vi "autocoupler_v2.vi"() -> ()   [LabVIEW 2018]
uses:
  coupler_state.ctl
  <userlib>/PDamp/gain.ctl
  <userlib>/stepper/velocity settings.ctl
  <userlib>/stepper/travel limits.ctl
  <userlib>/PDamp/channel.ctl
panel:
  in  "zpos":dbl(slide)=394.2760942760943 scale=-10.0..10.0
  in  "ypos":dbl(slide)=394.2760942760943 scale=-30.0..30.0
  in  "x_fine_stepper":dbl(slide)=-26.599326599326588 caption="x_fine" scale=-50.0..50.0
  in  "x_course_stepper":dbl(slide)=394.2760942760943 caption="x_course" min=100.0 max=3900.0 scale=100.0..3900.0
  out "saved postion":sgl[][](array[numeric]) format="%_7g"
  in  "save position":bool
  out "Coupled":dbl=7.033088235294118
  out "Stray":dbl=7.259191176470588
  out "stepper_z_pos":dbl=2218.076171875 caption="z"
  out "stepper_y_pos":dbl=1867.105712890625 caption="y"
  out "stepper_x_pos":dbl=367.677001953125 caption="x"
  in  "stop":bool
  in  "abort":bool
  out "Cam":bool
  out "PD":bool
  out "Steppers":bool
  out "Piezos":bool
  out "State":T1=enum."stop"
  in  "settings tabn":T2(tab)
  in  "optimization tab":enum32{"Nelder-Mead"}(tab)
  out "simplex area":sgl[](graph)=[0.375, 0.1875, 0.10546875, 0.29516602, 0.51086426, 1.6301422, 1.6301422, 0.40753555, 0.12771606, 0.04718399, 0.11667609, 0.068683326, 0.068683326, 0.1192682, 0.1192682, 0.1192682, 0.1192682, 0.1192682, 0.04766251, 0.028668227, 0.016006902, 0.010568131, 0.003405895, 0.0014921137, 0.0014921074, 0.0014921074, 0.00037302685]
  out "Coupled intensity":dbl[](graph)=[0.8621323529411764, 1.340073585510254, 1.340073585510254, 1.340073585510254, 1.4430147409439087, 1.566176414489746, 3.8327205181121826, 3.8327205181121826, 3.8327205181121826, 3.8327205181121826, 3.8327205181121826, 4.630514621734619, 4.630514621734619, 4.630514621734619, 5.512867450714111, 5.878676414489746, 6.665441036224365, 6.665441036224365, 6.878676414489746, 6.917279243469238, 6.917279243469238, 6.954044342041016, 6.966911792755127, 6.966911792755127, 6.998161792755127, 7.042279243469238, 7.042279243469238, 7.042279243469238]
  out "current iteration":i32=26
  in  "settling time[ms]":u32=200
  in  "contraction/expansion\nparameters":T3={"expansion coefficient"=2.0, "contraction coefficient"=0.5, "shrink coefficient"=0.5}
  in  "max iterations":i32=100
  out "avpos":cluster{sgl[], sgl[]}(graph)
  in  "initial simplex":T4={"Initial size y[µm]"=3.0, "Initial size z[µm]"=1.0}
  in  "termination size":sgl=0.001
  out "ygrapg1":cluster{sgl[], dbl[]}(graph)={[1000.0, 1000.95215, 1003.7415, 1006.9983, 1011.278, 1016.626, 1022.976, 1030.3162, 1038.6584, 1048.0615, 1058.5583, 1069.9756, 1082.6392, 1096.0486, 1110.4932, 1126.0901, 1142.0935, 1157.992, 1174.0125, 1190.2563, 1206.1584, 1221.9861, 1238.031, 1253.8794, 1270.1099, 1286.2317, 1302.4512, 1318.0383, 1334.093, 1350.0513, 1365.9436, 1381.9299, 1397.8223, 1413.9478, 1429.79, 1445.7373, 1461.737, 1477.8247, 1493.9551, 1509.7705, 1525.6897, 1541.8323, 1557.688, 1573.7183, 1589.8083, 1605.7129, 1621.8115, 1637.948, 1653.5559, 1669.6423, 1685.6653, 1701.6772, 1717.7258, 1733.6426, 1749.9048, 1765.6921, 1782.0288, 1797.8796, 1814.0698, 1829.7119, 1845.8142, 1861.7993, 1878.0872, 1893.6365, 1909.729, 1925.6506, 1941.6064, 1957.5867, 1973.6548, 1989.5972, 2005.3746, 2021.6052, 2037.6587, 2053.5632, 2069.4531, 2085.6738, 2101.5442, 2117.5244, 2133.617, 2149.5447, 2165.3137, 2181.8408, 2197.472, 2213.3643, 2229.3225, 2245.404, 2261.4014, 2277.3328, 2293.385, 2309.4397, 2325.315, 2341.5076, 2357.2522, 2373.4534, 2389.6082, 2405.2454, 2421.432, 2437.317, 2453.0212, 2469.2456, 2485.2368, 2501.0999, 2517.0715, 2533.2825, 2549.159, 2565.0476, 2581.0107, 2596.8494, 2613.0505, 2628.894, 2645.0586, 2661.001, 2676.9934, 2692.8577, 2708.8953, 2724.795, 2741.2122, 2756.858, 2772.865, 2788.9014, 2804.7375, 2820.7458, 2836.7175, 2852.915, 2868.7244, 2884.5178, 2899.3396, 2913.424, 2926.0327, 2937.7893, 2948.5083, 2958.5083, 2966.9885, 2974.7607, 2981.333, 2987.0557, 2991.665, 2995.2612, 2997.8699, 2999.4556], [7.983455882352941, 7.9724264705882355, 7.948529411764706, 7.9099264705882355, 7.849264705882353, 7.783088235294118, 7.735294117647059, 7.731617647058823, 7.825367647058823, 8.001838235294118, 8.117647058823529, 8.060661764705882, 8.084558823529411, 8.314338235294118, 8.625, 8.5, 8.472426470588236, 8.466911764705882, 8.465073529411764, 8.463235294117647, 8.461397058823529, 8.485294117647058, 8.492647058823529, 8.505514705882353, 8.439338235294118, 8.380514705882353, 8.306985294117647, 8.15625, 7.954044117647059, 7.783088235294118, 7.731617647058823, 7.762867647058823, 7.7849264705882355, 7.645220588235294, 7.610294117647059, 7.47610294117647, 7.161764705882353, 6.790441176470588, 6.492647058823529, 6.301470588235294, 6.1599264705882355, 6.1911764705882355, 6.080882352941177, 5.658088235294118, 5.461397058823529, 5.0036764705882355, 4.075367647058823, 3.0588235294117645, 2.0643382352941178, 1.349264705882353, 0.9172794117647058, 0.65625, 0.5110294117647058, 0.4411764705882353, 0.40625, 0.3860294117647059, 0.3676470588235294, 0.3676470588235294, 0.33088235294117646, 0.3290441176470588, 0.33455882352941174, 0.34191176470588236, 0.3639705882352941, 0.40808823529411764, 0.5588235294117647, 0.4430147058823529, 0.4944852941176471, 0.5422794117647058, 0.6213235294117647, 0.8088235294117647, 1.2610294117647058, 2.145220588235294, 3.6966911764705883, 5.827205882352941, 8.349264705882353, 10.806985294117647, 12.606617647058822, 13.707720588235293, 14.474264705882353, 15.262867647058822, 16.009191176470587, 16.470588235294116, 16.795955882352942, 17.18198529411765, 17.490808823529413, 17.626838235294116, 17.797794117647058, 18.020220588235293, 18.110294117647058, 18.198529411764707, 18.34375, 18.43566176470588, 18.441176470588236, 18.49448529411765, 18.49264705882353, 18.450367647058822, 18.43198529411765, 18.36764705882353, 18.314338235294116, 18.28125, 18.21875, 18.18014705882353, 18.176470588235293, 18.141544117647058, 18.11764705882353, 18.090073529411764, 18.097426470588236, 18.08639705882353, 18.051470588235293, 18.049632352941178, 18.06801470588235, 18.08639705882353, 18.112132352941178, 18.13051470588235, 18.143382352941178, 18.15441176470588, 18.15625, 18.159926470588236, 18.16360294117647, 18.178308823529413, 18.125, 18.115808823529413, 18.110294117647058, 18.080882352941178, 18.06801470588235, 18.064338235294116, 18.06801470588235, 18.080882352941178, 18.095588235294116, 18.10110294117647, 18.104779411764707, 18.106617647058822, 18.108455882352942, 18.14889705882353, 18.172794117647058, 18.176470588235293, 18.18014705882353, 18.183823529411764, 18.18198529411765, 18.18566176470588]}
  in  "initial_align":bool
  in  "z_scan_params":T5={"-offset"=100.0, "+offset"=500.0, "speed"=0.05, "threshold"=4.0, "y-offset"=0.0}
  in  "scan_y_params":T6={"startPos"=1000.0, "endPos"=3000.0, "speed"=1.0, "threshold"=1.0} {"endPos" min=0 max=4000; "startPos" min=0 max=4000}
  out "ygraph2":cluster{sgl[], dbl[]}(graph)={[1685.6653, 1686.499, 1688.3215, 1691.1292, 1694.1357, 1697.3169, 1700.5322, 1704.1016, 1708.3813, 1713.4692, 1716.6699, 1719.8682, 1723.0444, 1726.2427, 1729.4495, 1732.5269, 1735.697, 1738.8977, 1742.3877, 1745.6311, 1748.7732, 1751.9434, 1755.1404, 1758.3447, 1761.2573, 1764.436, 1767.6306, 1770.8411, 1774.0405, 1777.2473, 1780.6677, 1783.8635, 1787.0642, 1790.2393, 1793.479, 1796.676, 1799.6301, 1802.8064, 1806.0144, 1809.6118, 1812.815, 1815.9985, 1820.2808, 1825.3357, 1828.5254, 1831.7236, 1834.7595, 1837.959, 1841.1719, 1844.6936, 1847.8674, 1851.0742, 1854.2603, 1857.4609, 1860.6201, 1863.5168, 1866.7432, 1869.9121, 1874.6008, 1879.5203, 1882.9688, 1886.1768, 1889.3848, 1892.5635, 1895.7739, 1898.9429, 1901.8823, 1905.0769, 1908.2776, 1911.5027, 1914.685, 1917.8589, 1921.0779, 1924.646, 1928.9673, 1934.0332, 1937.2205, 1940.2246, 1943.4375, 1946.637, 1950.1782, 1954.602, 1959.751, 1962.9431, 1965.8203, 1969.0149, 1972.2168, 1975.4163, 1978.6108, 1981.8384, 1985.2454, 1987.7124, 1989.1687], [8.908088235294118, 8.935661764705882, 8.970588235294118, 8.996323529411764, 8.79595588235294, 8.994485294117647, 9.262867647058824, 9.323529411764707, 9.196691176470589, 9.384191176470589, 9.134191176470589, 9.169117647058824, 8.48345588235294, 8.503676470588236, 8.98345588235294, 9.20220588235294, 9.806985294117647, 10.07720588235294, 10.033088235294118, 10.148897058823529, 10.196691176470589, 10.238970588235293, 10.193014705882353, 10.1875, 10.13970588235294, 10.134191176470589, 10.126838235294118, 10.136029411764707, 10.169117647058824, 10.266544117647058, 10.373161764705882, 10.488970588235293, 10.680147058823529, 10.775735294117647, 10.85845588235294, 10.904411764705882, 10.875, 10.726102941176471, 10.455882352941176, 10.04595588235294, 9.220588235294118, 8.415441176470589, 7.50735294117647, 6.466911764705882, 5.525735294117647, 4.7775735294117645, 3.9301470588235294, 3.332720588235294, 2.625, 2.422794117647059, 2.4761029411764706, 3.0386029411764706, 2.479779411764706, 2.5533088235294117, 3.7279411764705883, 3.8731617647058822, 3.9871323529411766, 4.261029411764706, 5.665441176470588, 7.85110294117647, 9.647058823529411, 11.189338235294118, 13.503676470588236, 14.92095588235294, 17.13235294117647, 18.18014705882353, 19.69301470588235, 20.227941176470587, 21.159926470588236, 21.36948529411765, 21.641544117647058, 21.626838235294116, 21.360294117647058, 21.051470588235293, 20.65073529411765, 20.207720588235293, 19.996323529411764, 19.88051470588235, 19.81985294117647, 19.81066176470588, 19.84926470588235, 19.983455882352942, 20.06801470588235, 20.1875, 20.170955882352942, 20.11948529411765, 20.027573529411764, 19.928308823529413, 19.823529411764707, 19.68566176470588, 19.597426470588236, 19.509191176470587, 19.479779411764707]}
  out "zgraph":cluster{sgl[], dbl[]}(graph)={[2142.5427, 2143.4863, 2144.281, 2145.0757, 2145.8716, 2146.6602, 2147.4707, 2148.2068, 2149.0112, 2149.8047, 2150.5933, 2151.3916, 2152.1948, 2152.9944, 2153.7927, 2154.5813, 2155.3857, 2156.1816, 2156.98, 2157.782, 2158.5815, 2159.3774, 2160.2686, 2161.0657, 2161.8652, 2162.9053, 2163.7036, 2164.497, 2165.3088, 2166.0999, 2166.8933, 2167.6953, 2168.4949, 2169.292, 2170.094, 2170.8984, 2171.6907, 2172.5012, 2173.2947, 2174.0894, 2174.889, 2175.6982, 2176.488, 2177.295, 2178.0872, 2178.8953, 2179.6838, 2180.4968, 2181.7615, 2182.5537, 2183.3557, 2184.1516, 2184.95, 2185.8423, 2186.599, 2187.3462, 2188.2385, 2189.0369, 2189.8352, 2190.89, 2192.146, 2192.948, 2193.7402, 2194.535, 2195.4224, 2196.2134, 2196.958, 2198.0737, 2199.3347, 2200.1343, 2200.9424, 2201.7346, 2202.5317, 2203.335, 2204.1907, 2204.995, 2205.797, 2206.5967, 2207.384, 2208.186, 2208.933, 2209.735, 2210.536, 2211.3318, 2212.223, 2213.0322, 2213.8257, 2214.6155, 2215.4236, 2216.1328, 2216.9214, 2218.0762], [26.39889705882353, 26.501838235294116, 26.566176470588236, 26.488970588235293, 26.5, 26.46875, 26.422794117647058, 26.52941176470588, 26.393382352941178, 26.308823529411764, 26.386029411764707, 26.33639705882353, 26.43566176470588, 26.483455882352942, 26.308823529411764, 26.356617647058822, 26.338235294117645, 26.330882352941178, 26.488970588235293, 26.358455882352942, 26.3125, 26.463235294117645, 26.419117647058822, 26.551470588235293, 26.454044117647058, 26.27941176470588, 26.369485294117645, 26.31801470588235, 26.420955882352942, 26.47426470588235, 26.240808823529413, 26.33639705882353, 26.27389705882353, 26.220588235294116, 26.28676470588235, 26.03676470588235, 25.94485294117647, 26.165441176470587, 26.06801470588235, 26.209558823529413, 26.19301470588235, 25.863970588235293, 26.090073529411764, 26.169117647058822, 26.266544117647058, 26.387867647058822, 26.020220588235293, 26.06066176470588, 26.323529411764707, 26.159926470588236, 26.240808823529413, 25.928308823529413, 25.983455882352942, 26.28860294117647, 26.0625, 26.09191176470588, 25.71139705882353, 25.441176470588236, 25.753676470588236, 25.431985294117645, 25.53676470588235, 24.981617647058822, 25.18566176470588, 25.41360294117647, 24.875, 24.946691176470587, 24.71691176470588, 24.60110294117647, 25.290441176470587, 24.928308823529413, 25.544117647058822, 25.137867647058822, 25.270220588235293, 26.06985294117647, 25.21139705882353, 25.733455882352942, 25.884191176470587, 25.207720588235293, 27.90625, 26.965073529411764, 24.926470588235293, 28.25, 26.625, 24.78125, 22.27941176470588, 15.957720588235293, 16.490808823529413, 19.59191176470588, 17.606617647058822, 12.955882352941176, 8.367647058823529, 3.6011029411764706]}
  out "y_out":sgl=1837.1057
  out "z_out":sgl=2218.0762
  in  "stepsize x":i32
  in  "HWSerialNum x":i32=90897056 caption="serial nr"
  in  "HWSerialNum y":i32=90897057 caption="serial nr"
  in  "HWSerialNum z":i32=90897058 caption="serial nr"
  in  "MG17Motor y":refnum<k7>(container)
  in  "MG17Motor x":refnum<k7>(container)
  in  "MG17Motor z":refnum<k7>(container)
  in  "z_0":dbl=394.2760942760943 caption="z0" min=100.0 max=3900.0
  in  "y_0":dbl=394.2760942760943 caption="y0" min=100.0 max=3900.0
  in  "piezo_z_setmiddle":bool
  in  "piezo_y_setmiddle":bool
  in  "piezo_x_setmiddle":bool
  in  "x-axis":refnum<k7>(container)
  in  "y-axis":refnum<k7>(container)
  in  "z-axis":refnum<k7>(container)
  in  "serial number x":i32=91897094 caption="serial nr"
  in  "srl nr y-axis":i32=91897095 caption="serial nr"
  in  "srl nr z-axis":i32=91897096 caption="serial nr"
  in  "Change_cam_settings":bool
  out "Cam Info":T7={"Model"="IDS GmbH", "Camera ID"="UI124xSE-M", "Firmware"=""}
  in  "Camera ID":i32
  in  "Exposure[ms]":dbl=9.999750247413404 format="%#_13g"
  in  "camera live":bool=TRUE
  in  "ROI":T8={"posX"=0, "posY"=0, "Width"=1280, "height"=1024}
  out "ROI_current":T8
  in  "PD_comport":refnum<visa-resource-name>="COM4"
  out "status":string="rdy\r\n"
  in  "gain":T9=enum."1"
  in  "optimize":bool
  in  "stepper_home":bool
  in  "piezo_home":bool
  out "image":u8[][](graph)
  # "current position"
  # "x-axis"
  # "y-axis"
  # "z-axis"
  # "x-axis"
  # "y-axis"
  # "z-axis"
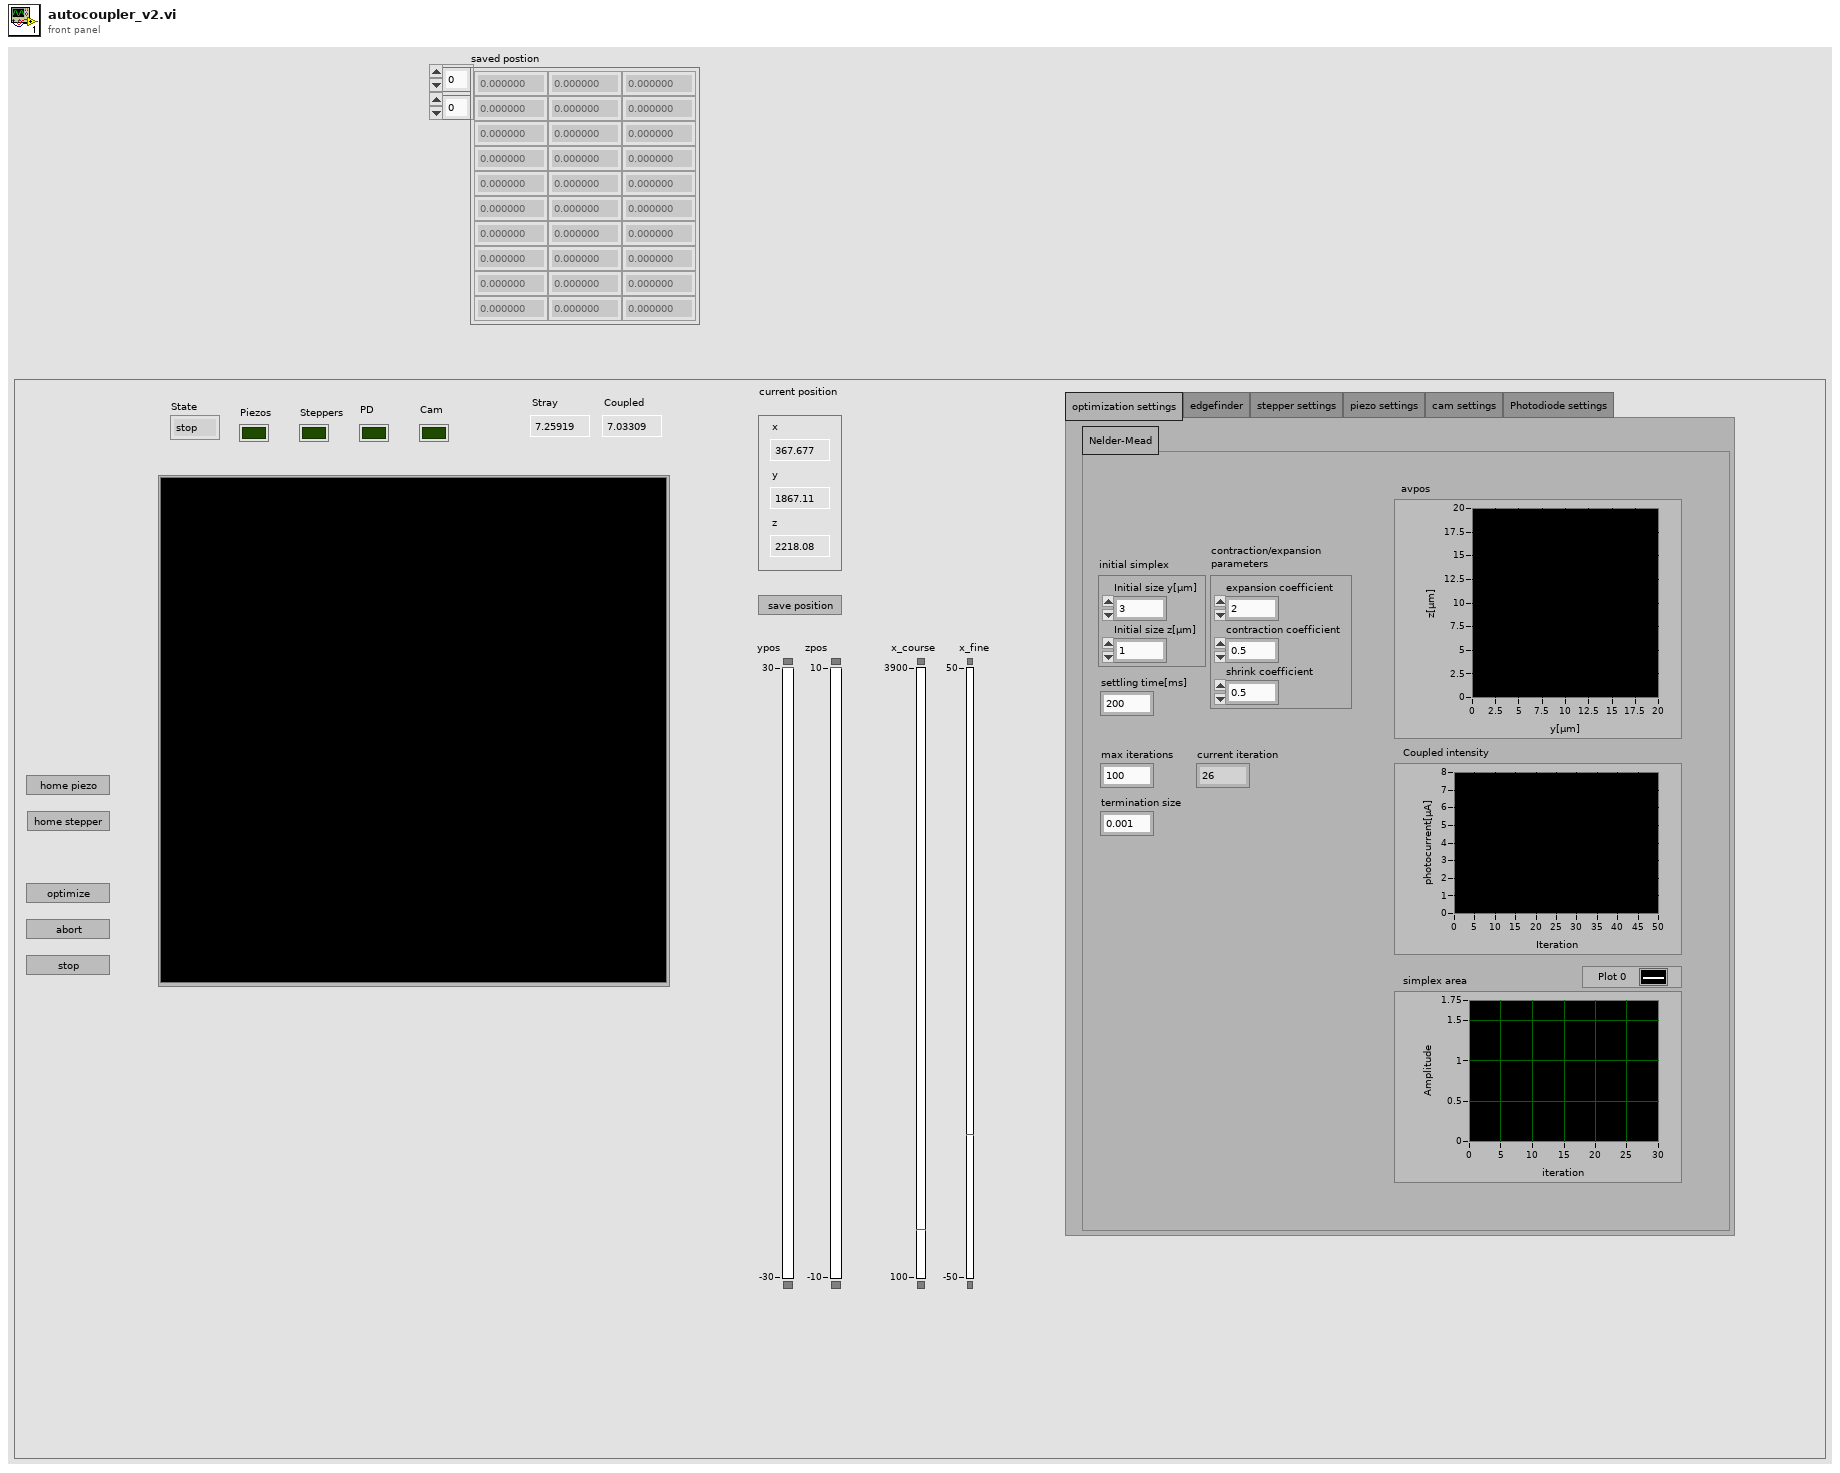
[diagram p1: front panel]
types:
  T1 = typedef "coupler_state.ctl" = enum16{"init", "idle", "zero_steppers", "zero_piezo", "edge_find", "save_position", "optimize", "stop", "error"}
  T2 = enum32{"optimization settings", "edgefinder", "stepper settings", "piezo settings", "cam settings", "Photodiode settings"}
  T3 = cluster{"expansion coefficient":dbl, "contraction coefficient":dbl, "shrink coefficient":dbl}
  T4 = cluster{"Initial size y[µm]":sgl, "Initial size z[µm]":sgl}
  T5 = cluster{"-offset":sgl, "+offset":sgl, "speed":sgl, "threshold":dbl, "y-offset":dbl}
  T6 = cluster{"startPos":sgl, "endPos":sgl, "speed":sgl, "threshold":sgl}
  T7 = cluster{"Model":string, "Camera ID":string, "Firmware":string}
  T8 = cluster{"posX":i32, "posY":i32, "Width":i32, "height":i32}
  T9 = typedef "gain.ctl" = enum16{"2/3", "1", "2", "4", "8", "16"}
  T10 = typedef "velocity settings.ctl" = cluster{"pfMinVel":sgl, "pfAccn":sgl, "pfMaxVel":sgl}
  T11 = typedef "channel.ctl" = enum16{"ch1", "ch2", "ch3", "ch4"}
  T12 = typedef "travel limits.ctl" = cluster{"pfRevPosLimit":sgl, "pfFwdPosLimit":sgl, "plLimitMode":i32}
  T13 = typedef "PDref.ctl" = cluster{"PD Reference":refnum<visa-resource-name>, "conversrion gain":dbl}
  T14 = cluster{"reference out":refnum<k7>, "reference out":refnum<k7>, "reference out":refnum<k7>}
  T15 = cluster{"reference out":refnum<k24>, "PDcluster":T13, cluster{"reference out":refnum<k7>, "reference out":refnum<k7>, "reference out":refnum<k7>}, cluster{"reference out":refnum<k7>, "reference out":refnum<k7>, "reference out":refnum<k7>}}
  T16 = cluster{"Reflected":sgl[][], "Expanded":sgl[][], "Contracted inside":sgl[][], "Contracted outside":sgl[][], "Shrunk":sgl[][]}
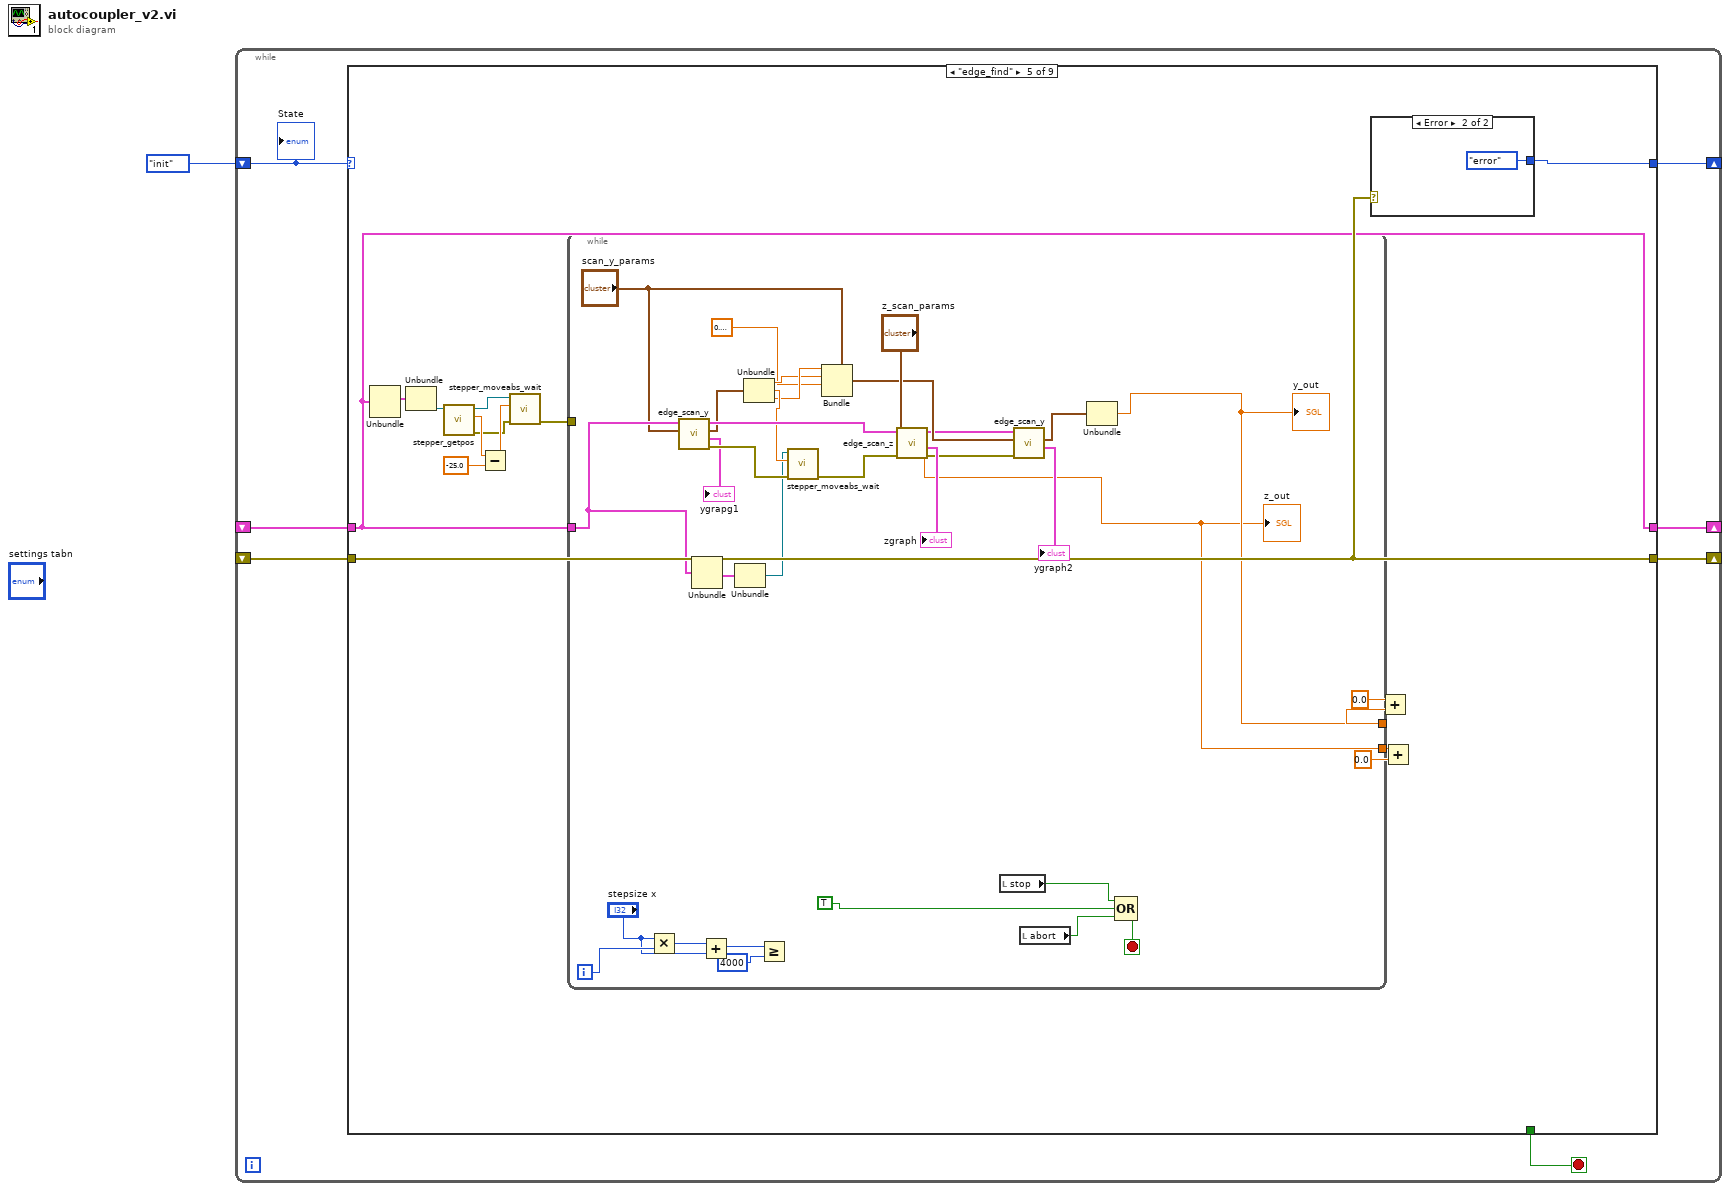
[diagram p0: block diagram]
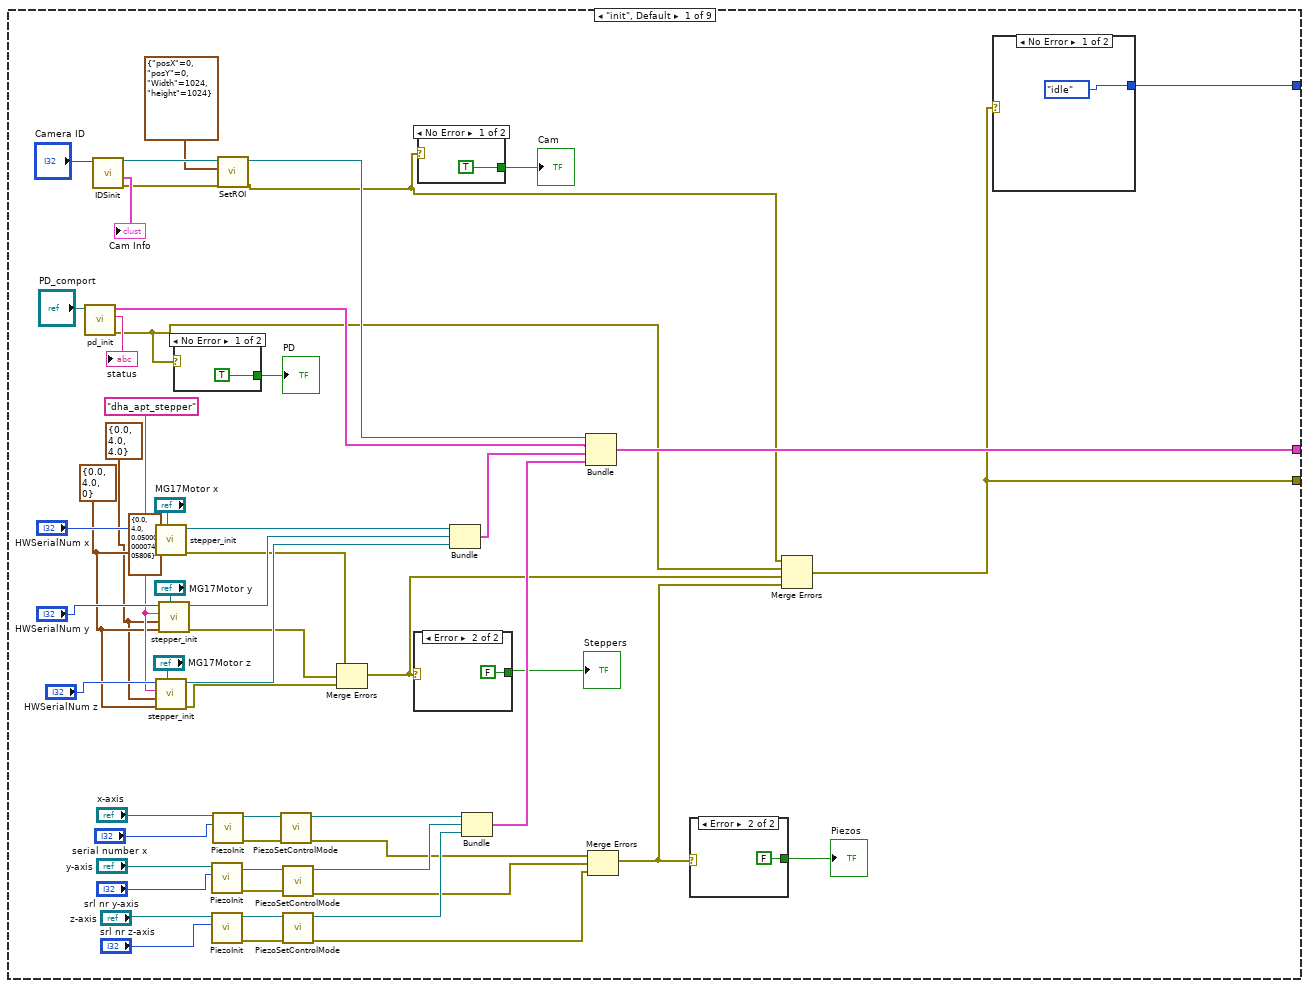
[diagram p2: hidden frame]
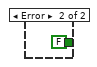
[diagram p3: hidden frame]
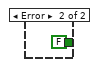
[diagram p4: hidden frame]
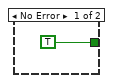
[diagram p5: hidden frame]
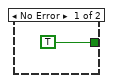
[diagram p6: hidden frame]
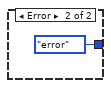
[diagram p7: hidden frame]
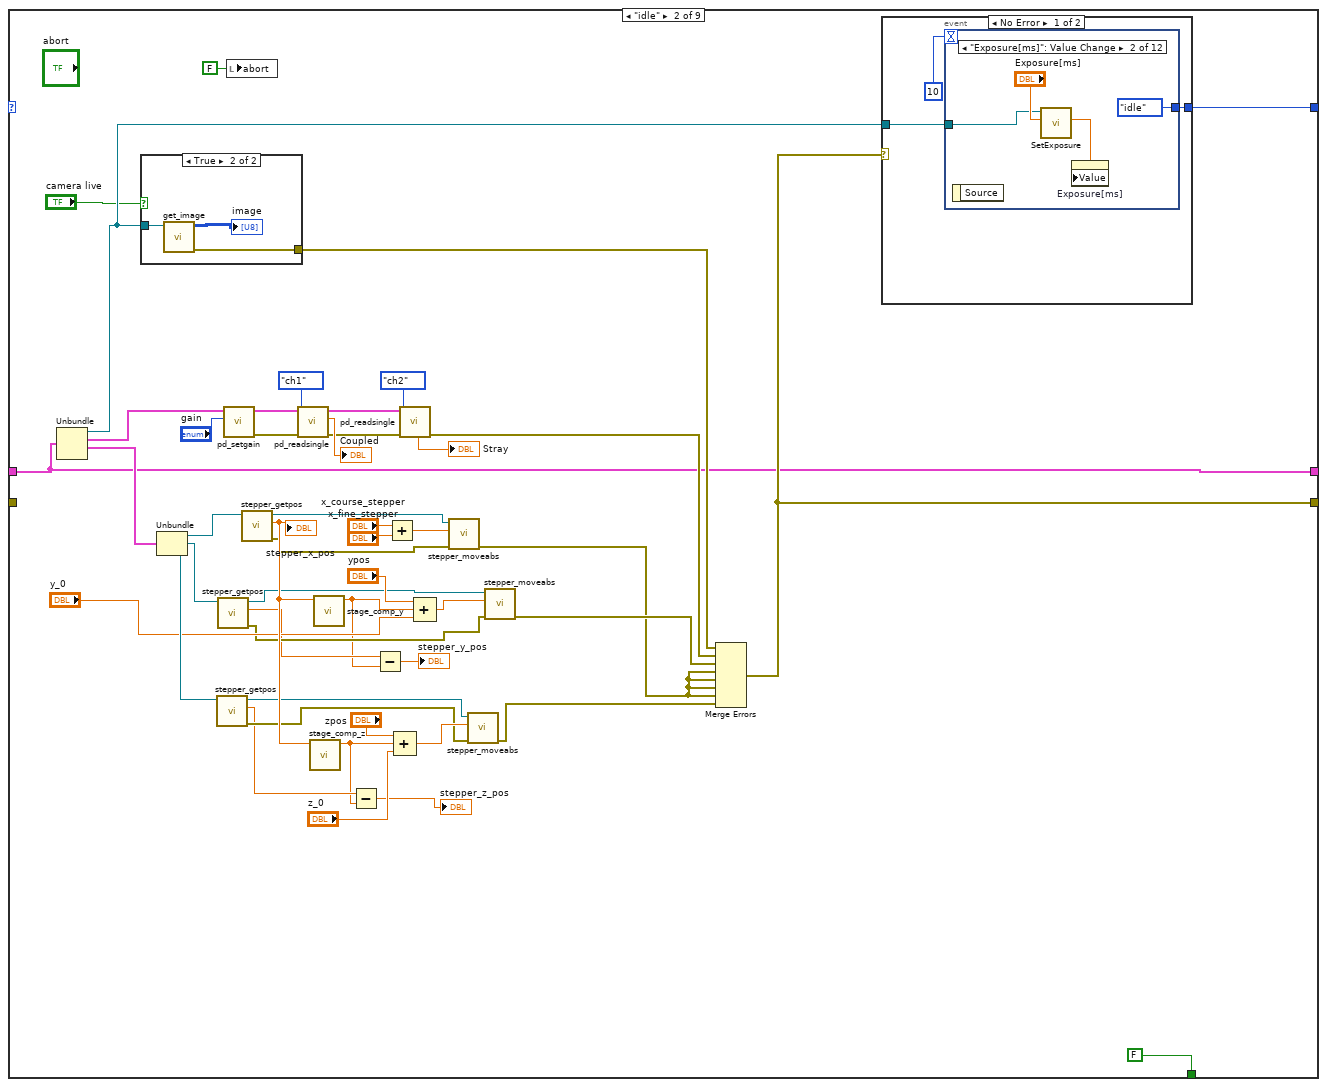
[diagram p8: hidden frame]
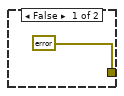
[diagram p9: hidden frame]
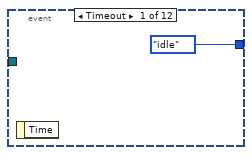
[diagram p10: hidden frame]
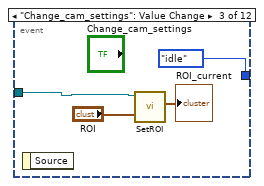
[diagram p11: hidden frame]
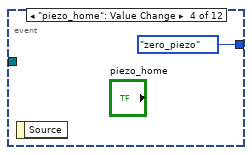
[diagram p12: hidden frame]
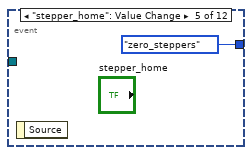
[diagram p13: hidden frame]
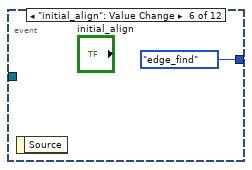
[diagram p14: hidden frame]
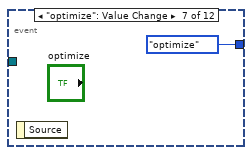
[diagram p15: hidden frame]
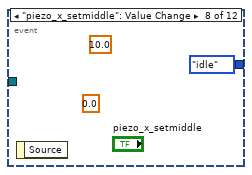
[diagram p16: hidden frame]
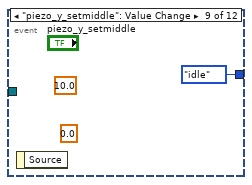
[diagram p17: hidden frame]
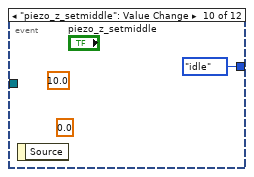
[diagram p18: hidden frame]
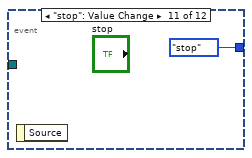
[diagram p19: hidden frame]
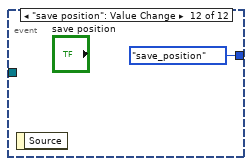
[diagram p20: hidden frame]
diagram:
  n1 = while {
    shift-right: [w7] -> _
    shift-left: coupler_state."init" -> [w8]
    shift-right: [w6] -> _
    shift-left: _ -> [w5]
    shift-right: [w3] -> _
    shift-left: _ -> [w2]
    stop <- w4 stop-if-true
    n2 = case shown="\"edge_find\"" w8 {
      tunnel: [w30 w122 w151 w170 w187 w245 w252 w318 w321] -> w7
      tunnel: [w31 w100 w150 w162 w185 w243 w251 w308 w331] -> w6
      tunnel: w5 -> [_ w100 w150 w162 w185 w243 w251 w308 w331]
      tunnel: [_ FALSE _ _ _ _ _ TRUE _] -> w4
      tunnel: [w11 w106 w149 w161 w186 w244 w249 w306 w322] -> w3
      tunnel: w2 -> [_ _ _ _ w186 w244 w250 w306 w323]
      frame "init", Default {
        w42 = T12 {"pfRevPosLimit"=0.0, "pfFwdPosLimit"=4.0, "plLimitMode"=0} ("travel limits")
        w10 = T10 {"pfMinVel"=0.0, "pfAccn"=4.0, "pfMaxVel"=4.0} ("velocity parameters")
        w43 = "dha_apt_stepper" ("parameter set")
        n3 = call <userlib>:"pd_init.vi"("VISA resource name"="PD_comport") -> ("error out"=w13:errorcluster, "status"=→"status":string, "PDcluster"=w32:T13)  [unwired: 8 in]
        n4 = call <userlib>:"IDSinit.vi"("Camera ID"="Camera ID") -> ("error out"=w17:errorcluster, "Cam Info"=→"Cam Info":T7, "reference out"=w29:refnum<k24>)  [unwired: 6 in, 1 out]
        n5 = call <userlib>:"stepper_init.vi"("MG17Motor"="MG17Motor x", "travel limits"=w42, "velocity parameters"=T10 {"pfMinVel"=0.0, "pfAccn"=4.0, "pfMaxVel"=0.05}, "parameter set"=w43, "HWSerialNum"="HWSerialNum x") -> ("error out"=w20:errorcluster, "reference out"=w39:refnum<k7>)  [unwired: 3 in, 2 out]
        n6 = call <userlib>:"stepper_init.vi"("MG17Motor"="MG17Motor z", "travel limits"=w42, "velocity parameters"=w10, "parameter set"=w43, "HWSerialNum"="HWSerialNum z") -> ("error out"=w22:errorcluster, "reference out"=w41:refnum<k7>)  [unwired: 3 in, 2 out]
        n7 = call <userlib>:"stepper_init.vi"("MG17Motor"="MG17Motor y", "travel limits"=w42, "velocity parameters"=w10, "parameter set"=w43, "HWSerialNum"="HWSerialNum y") -> ("error out"=w21:errorcluster, "reference out"=w40:refnum<k7>)  [unwired: 3 in, 2 out]
        n8 = case shown="No Error" w13 {
          tunnel: [TRUE ("Piezos") FALSE ("Piezos")] -> w18
          frame No Error {
          }
          frame Error {
          }
        }
        "PD" <- w18
        n9 = call <userlib>:"PiezoInit.vi"("reference"="y-axis", "HWSerialNum"="srl nr y-axis") -> ("reference out"=w56:refnum<k7>, "error out"=w54:errorcluster)  [unwired: 7 in]
        n10 = call <userlib>:"PiezoInit.vi"("reference"="z-axis", "HWSerialNum"="srl nr z-axis") -> ("reference out"=w57:refnum<k7>, "error out"=w53:errorcluster)  [unwired: 7 in]
        n11 = call <userlib>:"PiezoInit.vi"("reference"="x-axis", "HWSerialNum"="serial number x") -> ("reference out"=w58:refnum<k7>, "error out"=w55:errorcluster)  [unwired: 7 in]
        n12 = call <userlib>:"SetROI.vi"("error in (no error)"=w17, "SizeIn"=T8 {"posX"=0, "posY"=0, "Width"=1024, "height"=1024}, "reference in"=w29) -> ("error out"=w12:errorcluster, "reference out"=w27:refnum<k24>)  [unwired: 5 in, 1 out]
        n13 = call <userlib>:"PiezoSetControlMode.vi"("error in (no error)"=w55, "reference"=w58) -> ("error out"=w26:errorcluster, "reference out"=w50:refnum<k7>)  [unwired: 8 in]
        n14 = call <userlib>:"PiezoSetControlMode.vi"("error in (no error)"=w54, "reference"=w56) -> ("error out"=w25:errorcluster, "reference out"=w51:refnum<k7>)  [unwired: 8 in]
        n15 = call <userlib>:"PiezoSetControlMode.vi"("error in (no error)"=w53, "reference"=w57) -> ("error out"=w24:errorcluster, "reference out"=w52:refnum<k7>)  [unwired: 8 in]
        n16 = Merge Errors(w20, w21, w22) -> (w14:errorcluster)
        n17 = case shown="Error" w14 {
          tunnel: [TRUE ("Piezos") FALSE ("Piezos")] -> w19
          frame No Error {
          }
          frame Error {
          }
        }
        "Steppers" <- w19
        n18 = case shown="No Error" w12 {
          tunnel: [TRUE ("Piezos") FALSE ("Piezos")] -> w16
          frame No Error {
          }
          frame Error {
          }
        }
        "Cam" <- w16
        n19 = Bundle("reference out"=w39, "reference out"=w40, "reference out"=w41) -> (w33:T14)  [unwired: 1 in]
        n20 = Bundle("reference out"=w50, "reference out"=w51, "reference out"=w52) -> (w34:T14)  [unwired: 1 in]
        n21 = Bundle("reference out"=w27, "PDcluster"=w32, w33, w34) -> (w31:T15)  [unwired: 1 in]
        n22 = Merge Errors(w26, w25, w24) -> (w15:errorcluster)
        n23 = case shown="Error" w15 {
          tunnel: [TRUE ("Piezos") FALSE ("Piezos")] -> w23
          frame No Error {
          }
          frame Error {
          }
        }
        "Piezos" <- w23
        n24 = Merge Errors(w12, w13, w14, w15) -> (w11:errorcluster)
        n25 = case shown="No Error" w11 {
          tunnel: [coupler_state."idle" coupler_state."error"] -> w30
          frame No Error {
          }
          frame Error {
          }
        }
      }
      frame "idle" {
        n26 = Unbundle(w100) -> ("reference out"=w103:refnum<k24>, "PDcluster"=w121:T13, w110:T14)  [unwired: 1 out]
        n27 = case shown="True" "camera live" {
          tunnel: [errorcluster {"status"=FALSE, "code"=0, "source"=""} ("error out") w125] -> w104
          tunnel: w103 -> [_ w124]
          frame False {
          }
          frame True {
            n28 = call <userlib>:"get_image.vi"("reference"=w124) -> ("error out"=w125:errorcluster, "Array"=→"image":u8[][])  [unwired: 9 in]
          }
        }
        n29 = Unbundle(w110) -> ("reference out"=w113:refnum<k7>, "reference out"=w112:refnum<k7>, "reference out"=w111:refnum<k7>)
        n30 = call <userlib>:"stepper_getpos.vi"("reference"=w111) -> ("error out"=w85:errorcluster, "pfPosition[µm]"=w78:sgl, "reference out"=w91:refnum<k7>)  [unwired: 8 in]
        n31 = call <userlib>:"stepper_getpos.vi"("reference"=w112) -> ("error out"=w83:errorcluster, "pfPosition[µm]"=w76:sgl, "reference out"=w88:refnum<k7>)  [unwired: 8 in]
        n32 = call <userlib>:"pd_setgain.vi"("gain"="gain", "PDcluster in"=w121) -> ("error out"=w108:errorcluster, "PDcluster out"=w119:T13)  [unwired: 7 in, 1 out]
        n33 = local write "abort"(FALSE ("abort")) -> ()
        n34 = call <userlib>:"stepper_getpos.vi"("reference"=w113) -> ("error out"=w81:errorcluster, "pfPosition[µm]"=w95:sgl, "reference out"=w96:refnum<k7>)  [unwired: 8 in]
        "stepper_x_pos" <- w95
        n35 = call <userlib>:"pd_readsingle.vi"("PDcluster in"=w119, "channel"=channel."ch1", "error in (no error)"=w108) -> ("PDcluster out"=w117:T13, "photocurrent"=→"Coupled":dbl, "error out"=w107:errorcluster)  [unwired: 5 in]
        n36 = call "stage_comp_z.vi"("xpos"=w95) -> ("zcorr"=w77:dbl)  [unwired: 10 in]
        n37 = call "stage_comp_y.vi"("xpos"=w95) -> ("ycorr"=w75:dbl)  [unwired: 9 in, 1 out]
        n38 = Subtract(x=w78, y=w77) -> (x-y=→"stepper_z_pos":dbl)
        n39 = Subtract(x=w76, y=w75) -> (x-y=→"stepper_y_pos":dbl)
        n40 = Add(x="x_course_stepper", y="x_fine_stepper") -> (x+y=w97:dbl)
        n41 = Compound Arithmetic op=ADD("zpos", w77, "z_0") -> (w92:dbl)
        n42 = call <userlib>:"pd_readsingle.vi"("PDcluster in"=w117, "channel"=channel."ch2", "error in (no error)"=w107) -> ("photocurrent"=→"Stray":dbl, "error out"=w105:errorcluster)  [unwired: 5 in, 1 out]
        n43 = Compound Arithmetic op=ADD("ypos", w75, "y_0") -> (w79:dbl)
        n44 = call <userlib>:"stepper_moveabs.vi"("error in (no error)"=w81, "fAbsPos[µm]"=w97, "reference"=w96) -> ("error out"=w80:errorcluster)  [unwired: 7 in, 1 out]
        n45 = call <userlib>:"stepper_moveabs.vi"("error in (no error)"=w85, "fAbsPos[µm]"=w92, "reference"=w91) -> ("error out"=w84:errorcluster)  [unwired: 7 in, 1 out]
        n46 = call <userlib>:"stepper_moveabs.vi"("error in (no error)"=w83, "fAbsPos[µm]"=w79, "reference"=w88) -> ("error out"=w82:errorcluster)  [unwired: 7 in, 1 out]
        n47 = Merge Errors(w104, w105, w82, w80, w80, w80, w80, w84) -> (w106:errorcluster)
        n48 = case shown="No Error" w106 {
          tunnel: [w128 coupler_state."error"] -> w122
          tunnel: w103 -> [w127 _]
          frame No Error {
            n49 = event shown="[1] \"Exposure[ms]\": Value Change" {
              selector: _ -> [_ _ _ _ _ _ _ _ _ _ _ _]
              dyn-events: _ -> [_ _ _ _ _ _ _ _ _ _ _ _]
              timeout: 10 -> [_ _ _ _ _ _ _ _ _ _ _ _]
              tunnel: [coupler_state."idle" coupler_state."idle" coupler_state."idle" coupler_state."zero_piezo" coupler_state."zero_steppers" coupler_state."edge_find" coupler_state."optimize" coupler_state."idle" coupler_state."idle" coupler_state."idle" coupler_state."stop" coupler_state."save_position"] -> w128
              tunnel: w127 -> [_ w132 w137 _ _ _ _ _ _ _ _ _]
              event Timeout {
                n50 = event-data() -> ()  [unwired: 1 in, 1 out]
              }
              event "Exposure[ms]": Value Change {
                n51 = event-data() -> ()  [unwired: 1 in, 1 out]
                n52 = call <userlib>:"SetExposure.vi"("Exposure[ms]"="Exposure[ms]", "Reference in"=w132) -> ("exposure"=w133:dbl)  [unwired: 5 in, 3 out]
                n53 = property on="Exposure[ms]" class="DigNum (strict)"("Value"=w133) -> ()  [unwired: 2 in, 2 out]
              }
              event "Change_cam_settings": Value Change {
                n54 = event-data() -> ()  [unwired: 1 in, 1 out]
                n55 = call <userlib>:"SetROI.vi"("SizeIn"="ROI", "reference in"=w137) -> ("SizeOut"=→"ROI_current":T8)  [unwired: 6 in, 2 out]
              }
              event "piezo_home": Value Change {
                n56 = event-data() -> ()  [unwired: 1 in, 1 out]
              }
              event "stepper_home": Value Change {
                n57 = event-data() -> ()  [unwired: 1 in, 1 out]
              }
              event "initial_align": Value Change {
                n58 = event-data() -> ()  [unwired: 1 in, 1 out]
              }
              event "optimize": Value Change {
                n59 = event-data() -> ()  [unwired: 1 in, 1 out]
              }
              event "piezo_x_setmiddle": Value Change {
                (unwired) 0.0 ("z_fine_piezo")
                (unwired) 10.0 ("x_course_piezo")
                n60 = event-data() -> ()  [unwired: 1 in, 1 out]
              }
              event "piezo_y_setmiddle": Value Change {
                (unwired) 0.0 ("y_fine_piezo")
                (unwired) 10.0 ("y_course_piezo")
                n61 = event-data() -> ()  [unwired: 1 in, 1 out]
              }
              event "piezo_z_setmiddle": Value Change {
                (unwired) 0.0 ("z_fine_piezo")
                (unwired) 10.0 ("z_course_piezo")
                n62 = event-data() -> ()  [unwired: 1 in, 1 out]
              }
              event "stop": Value Change {
                n63 = event-data() -> ()  [unwired: 1 in, 1 out]
              }
              event "save position": Value Change {
                n64 = event-data() -> ()  [unwired: 1 in, 1 out]
              }
            }
          }
          frame Error {
          }
        }
      }
      frame "zero_steppers" {
        n65 = Unbundle(w150) -> (w158:T14)  [unwired: 3 out]
        n66 = Unbundle(w158) -> ("reference out"=w157:refnum<k7>, "reference out"=w156:refnum<k7>, "reference out"=w155:refnum<k7>)
        n67 = call <userlib>:"stepper_zero.vi"("reference"=w157) -> ("error out"=w152:errorcluster)  [unwired: 9 in, 1 out]
        n68 = call <userlib>:"stepper_zero.vi"("reference"=w156) -> ("error out"=w153:errorcluster)  [unwired: 9 in, 1 out]
        n69 = call <userlib>:"stepper_zero.vi"("reference"=w155) -> ("error out"=w154:errorcluster)  [unwired: 9 in, 1 out]
        n70 = Merge Errors(w152, w153, w154) -> (w149:errorcluster)
        n71 = case shown="Error" w149 {
          tunnel: [coupler_state."idle" coupler_state."error"] -> w151
          frame No Error {
          }
          frame Error {
          }
        }
      }
      frame "zero_piezo" {
        n72 = Unbundle(w162) -> (w169:T14)  [unwired: 3 out]
        n73 = Unbundle(w169) -> ("reference out"=w168:refnum<k7>, "reference out"=w167:refnum<k7>, "reference out"=w166:refnum<k7>)
        n74 = call <userlib>:"PiezoZeroAxis.vi"("reference"=w168) -> ("error out"=w163:errorcluster)  [unwired: 9 in, 1 out]
        n75 = call <userlib>:"PiezoZeroAxis.vi"("reference"=w167) -> ("error out"=w164:errorcluster)  [unwired: 9 in, 1 out]
        n76 = call <userlib>:"PiezoZeroAxis.vi"("reference"=w166) -> ("error out"=w165:errorcluster)  [unwired: 9 in, 1 out]
        n77 = Merge Errors(w163, w164, w165) -> (w161:errorcluster)
        n78 = case shown="Error" w161 {
          tunnel: [coupler_state."idle" coupler_state."error"] -> w170
          frame No Error {
          }
          frame Error {
          }
        }
      }
      frame "edge_find" {
        n79 = Unbundle(w185) -> (w184:T14)  [unwired: 3 out]
        n80 = Unbundle(w184) -> ("reference out"=w183:refnum<k7>)  [unwired: 2 out]
        n81 = call <userlib>:"stepper_getpos.vi"("reference"=w183) -> ("error out"=w177:errorcluster, "pfPosition[µm]"=w182:sgl, "reference out"=w179:refnum<k7>)  [unwired: 8 in]
        n82 = Subtract(x=w182, y=sgl -25.0) -> (x-y=w180:sgl)
        n83 = call <userlib>:"stepper_moveabs_wait.vi"("error in (no error)"=w177, "fAbsPos[µm]"=w180, "reference"=w179) -> ("error out"=w178:errorcluster)  [unwired: 7 in, 1 out]
        n84 = while {
          tunnel: w185 -> [w215]
          tunnel: [w190] -> w176
          tunnel: [w192] -> w174
          tunnel: w178 -> [_]
          i -> [w199]
          stop <- w217 stop-if-true
          n85 = Multiply(x="stepsize x", y=w199) -> (x*y=w191:i32)
          n86 = call "edge_scan_y.vi"("scan_y_params"="scan_y_params", "refs"=w215) -> ("error out"=w213:errorcluster, "graph"=→"ygrapg1":cluster{sgl[], dbl[]}, "result"=w205:cluster{"maxy":sgl, "midy":sgl, "miny":sgl}, "refs out"=w207:T15)  [unwired: 6 in]
          n87 = Unbundle(w215) -> (w214:T14)  [unwired: 3 out]
          n88 = Add(x=w191, y="stepsize x") -> (x+y=w197:i32)
          n89 = Unbundle(w214) -> ("reference out"=w193:refnum<k7>)  [unwired: 2 out]
          n90 = Unbundle(w205) -> ("maxy"=w202:sgl, "midy"=w204:sgl, "miny"=w203:sgl)
          n91 = Greater Or Equal?(x=w197, y=4000) -> ()  [unwired: 1 out]
          n92 = call <userlib>:"stepper_moveabs_wait.vi"("error in (no error)"=w213, "fAbsPos[µm]"=w204, "reference"=w193) -> ("error out"=w211:errorcluster)  [unwired: 7 in, 1 out]
          n93 = Bundle(cluster="scan_y_params", "startPos"=w203, "endPos"=w202, "speed"=sgl 0.2) -> (w195:T6)  [unwired: 1 in]
          n94 = call "edge_scan_z.vi"("error in (no error)"=w211, "z_scan_params"="z_scan_params", "refs"=w207) -> ("error out"=w208:errorcluster, "graph"=→"zgraph":cluster{sgl[], dbl[]}, "z_out"=w190:sgl, "refs out"=w188:T15)  [unwired: 4 in]
          "z_out" <- w190
          n95 = local read "stop"() -> (w216:bool)
          n96 = call "edge_scan_y.vi"("error in (no error)"=w208, "scan_y_params"=w195, "refs"=w188) -> ("graph"=→"ygraph2":cluster{sgl[], dbl[]}, "result"=w200:cluster{"maxy":sgl, "midy":sgl, "miny":sgl})  [unwired: 5 in, 2 out]
          n97 = local read "abort"() -> (w218:bool)
          n98 = Unbundle(w200) -> ("midy"=w192:sgl)  [unwired: 2 out]
          "y_out" <- w192
          n99 = Compound Arithmetic op=OR(w216, TRUE ("value"), w218) -> (w217:bool)
        }
        n100 = case shown="Error" w186 {
          tunnel: [coupler_state."idle" coupler_state."error"] -> w187
          frame No Error {
          }
          frame Error {
          }
        }
        n101 = Add(x=sgl 0.0, y=w174) -> ()  [unwired: 1 out]
        n102 = Add(x=w176, y=sgl 0.0) -> ()  [unwired: 1 out]
      }
      frame "save_position" {
        n103 = local read "stepper_x_pos"() -> (w224:dbl)
        n104 = local read "stepper_y_pos"() -> (w223:dbl)
        n105 = local read "stepper_z_pos"() -> (w222:dbl)
        n106 = Unbundle(w243) -> (w235:T14, w242:T14)  [unwired: 2 out]
        n107 = Unbundle(w242) -> ("reference out"=w241:refnum<k7>, "reference out"=w240:refnum<k7>, "reference out"=w239:refnum<k7>)
        n108 = Unbundle(w235) -> ("reference out"=w232:refnum<k7>, "reference out"=w233:refnum<k7>, "reference out"=w234:refnum<k7>)
        n109 = call <userlib>:"PiezoGetPosition.vi"("reference"=w239) -> ("Position"=w238:sgl)  [unwired: 4 in, 2 out]
        n110 = call <userlib>:"PiezoGetPosition.vi"("reference"=w241) -> ("Position"=w236:sgl)  [unwired: 4 in, 2 out]
        n111 = call <userlib>:"PiezoGetPosition.vi"("reference"=w240) -> ("Position"=w237:sgl)  [unwired: 4 in, 2 out]
        n112 = call <userlib>:"stepper_getpos.vi"("reference"=w232) -> ()  [unwired: 8 in, 3 out]
        n113 = call <userlib>:"stepper_getpos.vi"("reference"=w233) -> ()  [unwired: 8 in, 3 out]
        n114 = call <userlib>:"stepper_getpos.vi"("reference"=w234) -> ()  [unwired: 8 in, 3 out]
        n115 = Build Array(w236, w237, w238) -> (w231:sgl[])
        n116 = Build Array(w224, w223, w222) -> (w227:dbl[])
        n117 = Multiply(x=w227, y=1 ("pfPosition")) -> (x*y=w225:dbl[])
        n118 = Add(x=w225, y=w231) -> (x+y=w230:dbl[])
        n119 = feedback #1(dbl[][] []) -> (w228:dbl[][])
        n120 = Build Array (concatenate)(w228, w230) -> (w229:dbl[][])
        "saved postion" <- w229
        n121 = feedback-in #1(w229) -> ()
        n122 = case shown="No Error" w244 {
          tunnel: [coupler_state."idle" coupler_state."error"] -> w245
          frame No Error {
          }
          frame Error {
          }
        }
      }
      frame "optimize" {
        n123 = case shown="\"Nelder-Mead\", Default" "optimization tab" {
          tunnel: w251 -> [w265]
          tunnel: w250 -> [w266]
          tunnel: [w263] -> w249
          frame "Nelder-Mead", Default {
            n124 = local read "Coupled"() -> (w258:dbl)
            n125 = call "nelder_make_initial_simplex.vi"("error in (no error)"=w266, "settling time"="settling time[ms]", "initial simplex"="initial simplex", "References"=w265) -> ("error out"=w262:errorcluster, "output simplex"=w261:sgl[][])  [unwired: 4 in]
            n126 = property on="settings tabn" class="TabCtl (strict)"("Value"=T2."optimization settings" ("settings tabn")) -> (error out=w254:errorcluster)  [unwired: 2 in, 1 out]
            n127 = Multiply(x=w258, y=-1.0) -> (x*y=w257:dbl)
            n128 = Build Array(w257) -> (w259:dbl[])
            n129 = while {
              shift-right: [w302] -> w263
              shift-left: w262 -> [w299]
              tunnel: w265 -> [w268]
              tunnel: "settling time[ms]" -> [w301]
              shift-right: [w296] -> _
              shift-left: w261 -> [w298]
              shift-right: [w292] -> _
              shift-left: _ -> [w290]
              shift-right: [w291] -> _
              shift-left: _ -> [w287]
              shift-right: [w284] -> _
              shift-left: w259 -> [w285]
              shift-right: [w276] -> _
              shift-left: sgl[] [] -> [w277]
              tunnel: w254 -> [_]
              i -> [w295]
              stop <- w269 stop-if-true
              n130 = call "nelder_make_potential_simplexes.vi"("error in (no error)"=w299, "current simplex"=w298, "parameters"="contraction/expansion\nparameters") -> ("error out"=w278:errorcluster, "Output Simplexes"=w281:T16)  [unwired: 7 in]
              n131 = call "opt_fix_piezo_range_issue.vi"("error in"=w278, "Simplexes in"=w281, "references"=w268) -> ("error out"=w279:errorcluster, "simplexes out"=w267:T16, "references out"=w280:T15)  [unwired: 5 in, 1 out]
              n132 = call "nelder_make_next_simplex.vi"("error in"=w279, "settling time"=w301, "input \nsimplex"=w267, "refs"=w280) -> ("error out"=w302:errorcluster, "next simplex"=w294:sgl[][])  [unwired: 6 in]
              n133 = call "nelder_sort.vi"("input simplex"=w294) -> ("output simplex"=w296:sgl[][])  [unwired: 10 in]
              n134 = call "nelder_get_center_of_simplex.vi"("simplex input"=w294) -> ("area"=w275:sgl, "min"=w286:sgl, "z"=w288:sgl, "y"=w289:sgl)  [unwired: 7 in]
              n135 = local read "abort"() -> (w272:bool)
              n136 = Greater?(x=w295, y="max iterations") -> (0:w273:bool)
              n137 = Less?(x=w275, y="termination size") -> (x < y?=w270:bool)
              n138 = local read "stop"() -> (w271:bool)
              n139 = Build Array (concatenate)(w290, w289) -> (w292:sgl[])
              n140 = Build Array (concatenate)(w285, w286) -> (w284:dbl[])
              n141 = Build Array (concatenate)(w287, w288) -> (w291:sgl[])
              n142 = Build Array (concatenate)(w277, w275) -> (w276:sgl[])
              "simplex area" <- w276
              n143 = Multiply(x=w284, y=sgl -1.0 ("max")) -> (x*y=→"Coupled intensity":dbl[])
              n144 = Bundle(w292, w291) -> (→"avpos":cluster{sgl[], sgl[]})  [unwired: 1 in]
              n145 = Compound Arithmetic op=OR(w270, w271, w272, w273) -> (w269:bool)
              "current iteration" <- w295
            }
          }
        }
        n146 = case shown="Error" w249 {
          tunnel: [coupler_state."idle" coupler_state."error"] -> w252
          frame No Error {
          }
          frame Error {
          }
        }
      }
      frame "stop" {
        w305 = FALSE ("stop")
        n147 = Unbundle(w308) -> ("PDcluster"=w309:T13, w313:T14, w317:T14)  [unwired: 1 out]
        n148 = Unbundle(w313) -> ("reference out"=w310:refnum<k7>, "reference out"=w311:refnum<k7>, "reference out"=w312:refnum<k7>)
        n149 = Unbundle(w317) -> ("reference out"=w316:refnum<k7>, "reference out"=w315:refnum<k7>, "reference out"=w314:refnum<k7>)
        n150 = call <userlib>:"pd_close.vi"("PDcluster in"=w309) -> ()  [unwired: 10 in, 1 out]
        n151 = call <userlib>:"stepper_close.vi"("reference"=w310) -> ()  [unwired: 9 in, 2 out]
        n152 = call <userlib>:"stepper_close.vi"("reference"=w311) -> ()  [unwired: 9 in, 2 out]
        n153 = call <userlib>:"stepper_close.vi"("reference"=w312) -> ()  [unwired: 9 in, 2 out]
        n154 = call <userlib>:"PiezoClose.vi"("reference"=w316) -> ()  [unwired: 5 in, 2 out]
        n155 = call <userlib>:"PiezoClose.vi"("reference"=w315) -> ()  [unwired: 5 in, 2 out]
        n156 = call <userlib>:"PiezoClose.vi"("reference"=w314) -> ()  [unwired: 5 in, 2 out]
        n157 = local write "stop"(w305) -> ()
        n158 = local write "Steppers"(w305) -> ()
        n159 = local write "Piezos"(w305) -> ()
        n160 = local write "Cam"(w305) -> ()
        n161 = local write "PD"(w305) -> ()
        n162 = case shown="Error" w306 {
          tunnel: [coupler_state."stop" coupler_state."stop"] -> w318
          frame No Error {
          }
          frame Error {
          }
        }
      }
      frame "error" {
        n163 = Unbundle(w323) -> ("source"=w329:string)  [unwired: 2 out]
        n164 = Concatenate Strings("found error:" ("message"), w329, "continue or stop?" ("string")) -> (w327:string)
        n165 = Two Button Dialog(message=w327, 1:"stop" ("F button name (\"Cancel\")"), 2:"continue" ("T button name (\"OK\")")) -> (T button?=w324:bool)
        n166 = case shown="False" w324 {
          tunnel: w323 -> [w332 w336]
          tunnel: [w332 w335] -> w322
          tunnel: [coupler_state."stop" coupler_state."idle"] -> w321
          frame False {
          }
          frame True {
            n167 = call <vilib>:"Clear Errors.vi"("error in (no error)"=w336) -> ("error out"=w335:errorcluster)  [unwired: 5 in, 1 out]
          }
        }
      }
    }
    "State" <- w8
  }
